vi "Dequeue Message.vi"(8 "error in (no error)":errorcluster, 10 "timeout in ms (-1)":i32=-1, 11 "Message Queue":refnum<queue>) -> (0 "error out":errorcluster, 1 "Message Data":variant, 2 "Message":string, 3 "dup Message Queue":refnum<queue>, 4 "timed out?":bool)   [LabVIEW 2014, in "UI_ProgressDlg.lvlib" / "UI_ProgressDlg.lvclass"]
doc: "This VI pulls messages off the Message Queue. It has special error handling to account for an error occurring on the last iteration of the Message Handling Loop.\n\nNo Error - normal Dequeue Element operation.\nError - check if it is an error code we wish to ignore. If so, clear the error and perform a normal Dequeue Element. If not, output the error, and put a 'Stop' message on the Message Queue."
uses:
  UI_ProgressDlg.lvclass
  Message Cluster.ctl
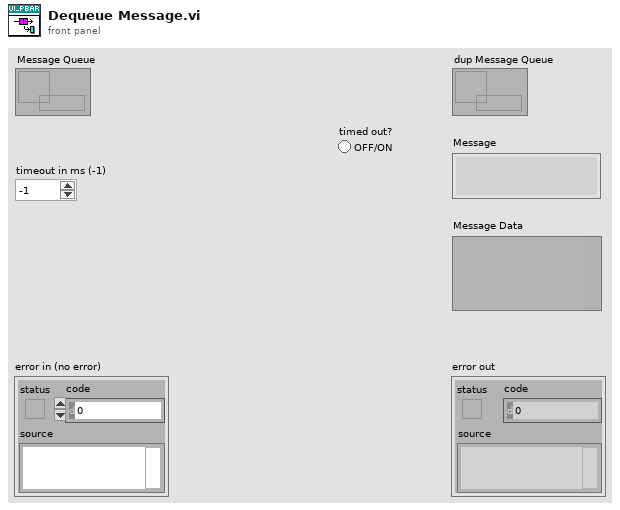
[diagram p1: front panel]
types:
  T1 = typedef "UI_ProgressDlg.lvlib/UI_ProgressDlg.lvclass/Message Cluster.ctl" = cluster{"Message":string, "Message Data":variant}
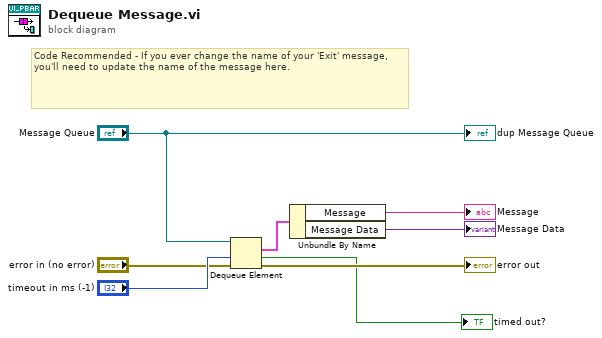
[diagram p0: block diagram]
diagram:
  # "Code Recommended - If you ever change the name of your 'Exit' message, you'll need to update the name of the message here."
  n1 = Dequeue Element(queue="Message Queue", timeout in ms (-1)="timeout in ms (-1)", error in (no error)="error in (no error)") -> (element=w1:T1, timed out?=→"timed out?":bool, error out=→"error out":errorcluster)  [unwired: 1 out]
  n2 = Unbundle By Name(w1) -> ("Message"=→"Message":string, "Message Data"=→"Message Data":variant)
  "dup Message Queue" <- "Message Queue"
